vi "write single relay.vi"(8 "error in (no error)":errorcluster, 9 "on/off":bool, 10 "index":i32, 11 "hardware in":refnum<class "hardware.lvclass">) -> (0 "error out":errorcluster, 3 "hardware out":refnum<class "hardware.lvclass">)   [LabVIEW 2025, in "hardware.lvclass"]
uses:
  hardware.lvclass
  hardware.lvclass/hardware.ctl
  <vilib>/DAQmx/write.llb/DAQmx Write (Digital 1D Bool NChan 1Samp 1Line).vi
  <vilib>/DAQmx/miscellaneous.llb/DAQmx Fill In Error Info.vi
panel:
  out "x-y":dbl
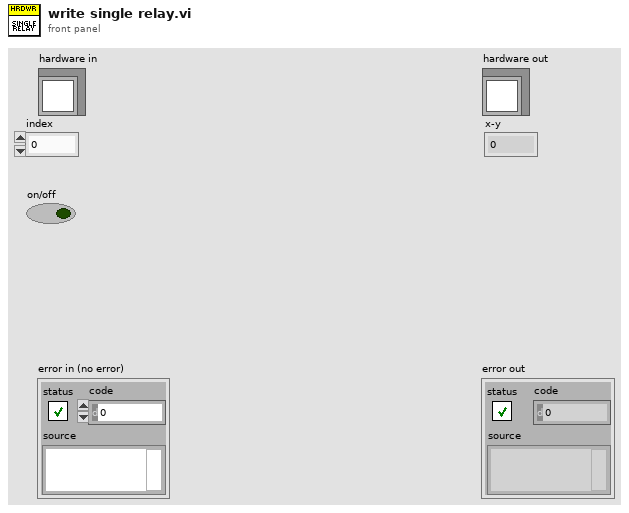
[diagram p1: front panel]
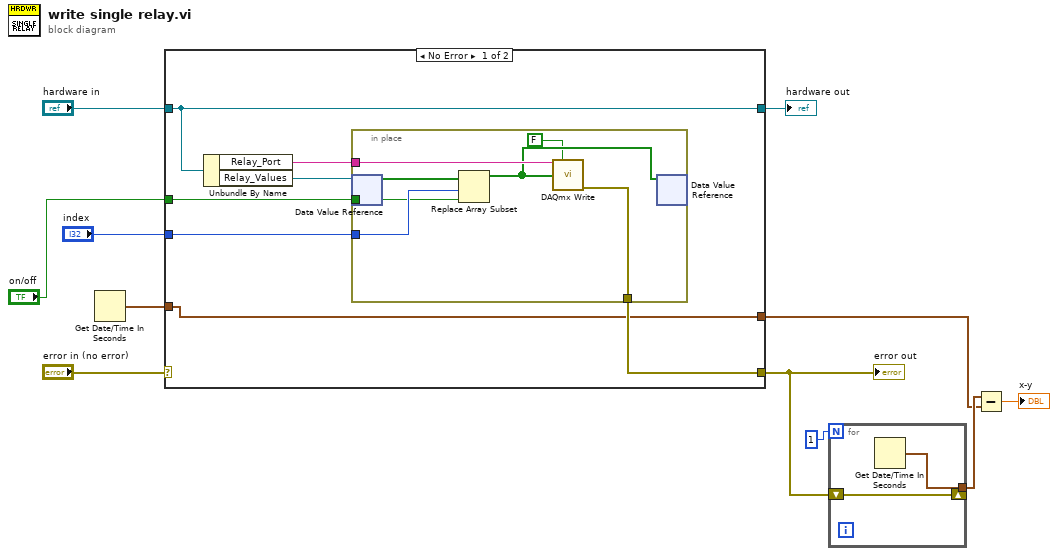
[diagram p0: block diagram]
diagram:
  n1 = Get Date/Time In Seconds() -> (seconds since 1Jan1904=w6:timestamp)
  n2 = case shown="No Error" "error in (no error)" {
    selector: "error in (no error)" -> [_ w26]
    tunnel: [w18 w27] -> w9
    tunnel: "hardware in" -> [w18 w27]
    tunnel: "index" -> [w15 _]
    tunnel: [w14 w26] -> w3
    tunnel: "on/off" -> [w13 _]
    tunnel: w6 -> [w12 _]
    tunnel: [w12 _] -> w1
    frame No Error {
      n3 = Unbundle By Name(w18) -> ("Relay_Port"=w16:string, "Relay_Values"=w17:refnum<data-value>)
      n4 = in-place {
        in-place-border: w16 -> [w23]
        in-place-border: w15 -> [w24]
        in-place-border: [w21] -> w14
        in-place-border: w13 -> [w20]
        n5 = in-place-dvr #1(w17) -> (w25:bool[])  [unwired: 1 out]
        n6 = Replace Array Subset(array=w25, new element=w20, index=w24) -> (w22:bool[])
        n7 = call-poly <vilib>:"DAQmx Write.vi"("task/channels in"=w23, "auto start"=FALSE, "data"=w22) -> ("error out"=w21:errorcluster)  [unwired: 10 in, 2 out]
        n8 = in-place-dvr #1(w22) -> ()  [unwired: 2 out]
      }
    }
    frame Error {
    }
  }
  "error out" <- w3
  "hardware out" <- w9
  n9 = for {
    N: 1 -> [_]
    tunnel: [w29] -> w2
    shift-right: [w28] -> _
    shift-left: w3 -> [w28]
    n10 = Get Date/Time In Seconds() -> (seconds since 1Jan1904=w29:timestamp)
  }
  n11 = Subtract(x=w2, y=w1) -> (x-y=→"x-y":dbl)
